vi "Teleop.vi"(10 "Match Info":T2={"Autonomous Elapsed Seconds"=0.0, "TeleOp Elapsed Seconds"=0.0, "Disabled Elapsed Seconds"=0.0, "Visited Autonomous"=FALSE, "Visited TeleOp"=FALSE, "Visited Disabled"=FALSE, "Autonomous Settings"={"Autonomous Style"=enum."Independent", "VI Refnum"=refnum}}, 11 "Call Context":T3) -> ()   [LabVIEW 2014]
doc: "This VI is called for each TeleOp packet received from the DS where the robot is not disabled. It is often used to read from the joysticks and update I/O or to update setpoints for timed control loops. It should complete and return within 20 milliseconds or it may miss DS packets."
uses:
  <vilib>/Rock Robotics/WPI/DriverStation/WPI_DriverStationDerivedRobotMode.ctl
  <vilib>/Rock Robotics/WPI/DriverStation/WPI_DriverStationMatch Info.ctl
  <vilib>/Rock Robotics/Network Tables/SD Read Boolean.vi
  <vilib>/Rock Robotics/Network Tables/SD Read Number.vi
  Robot Global Data.vi
  <vilib>/Rock Robotics/Network Tables/SD Write Numeric Array.vi
panel:
  out "Normalized Rect":T1
  out "Center":cluster{dbl, dbl}
  out "Applied Throttle":dbl
  out "Val":dbl
  out "RawVal":i32
  out "Stopped?":string
  out "Direction":string
  out "Distance":dbl
  out "Sample Slider 0":dbl(slide) scale=0.0..5.0
  out "Sample Boolean 1":bool
  out "Sample Boolean 0":bool
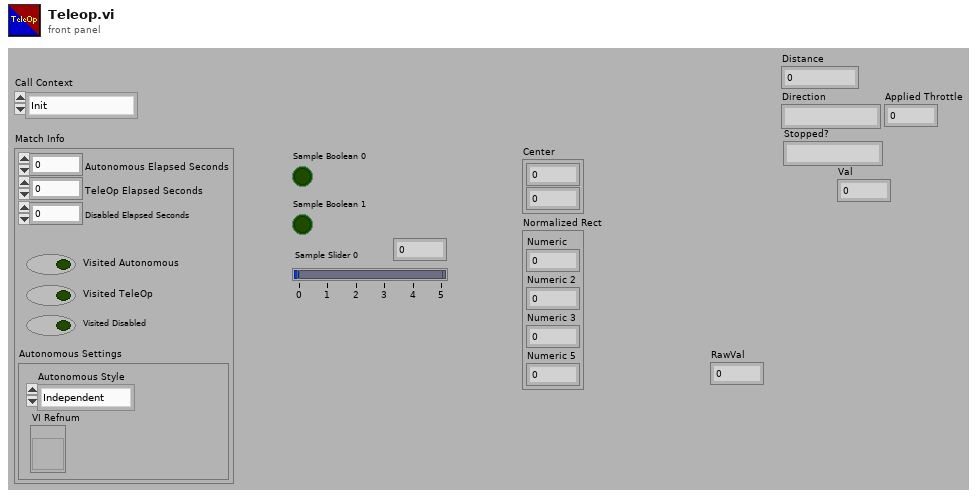
[diagram p1: front panel]
types:
  T1 = cluster{"Numeric":dbl, "Numeric 2":dbl, "Numeric 3":dbl, "Numeric 5":dbl}
  T2 = typedef "WPI_DriverStationMatch Info.ctl" = cluster{"Autonomous Elapsed Seconds":dbl, "TeleOp Elapsed Seconds":dbl, "Disabled Elapsed Seconds":dbl, "Visited Autonomous":bool, "Visited TeleOp":bool, "Visited Disabled":bool, "Autonomous Settings":cluster{"Autonomous Style":enum16{"Iterative", "Independent"}, "VI Refnum":refnum<vi>}}
  T3 = typedef "WPI_DriverStationDerivedRobotMode.ctl" = enum16{"Init", "Execute", "Stop"}
  T4 = typedef "WPI_MotorControlDeviceRef.ctl" = cluster{"DeviceStatus":errorcluster, "Type":T5, "PWM":cluster{"Controller":T6, "PWM Channel":T7, "DeadBand":T8}, "CAN":cluster{"Device Number":u8, "Control Mode":T9, "Semaphore":T10, "Max Vout":dbl, "TalonSRX Control Mode":T11}, "Invert":bool, "TransformRef":T12, "InvTransformRef":T12}
  T5 = typedef "WPI_MotorControlType.ctl" = enum16{"PWM", "CAN", "CANTalonSRX"}
  T6 = typedef "FPGA_TypedefDigitalModule.ctl" = enum16{"Controller 1"}
  T7 = typedef "FPGA_DIOPWMChannel.ctl" = enum8{"PWM 0", "PWM 1", "PWM 2", "PWM 3", "PWM 4", "PWM 5", "PWM 6", "PWM 7", "PWM 8", "PWM 9", "PWM MXP 0", "PWM MXP 1", "PWM MXP 2", "PWM MXP 3", "PWM MXP 4", "PWM MXP 5", "PWM MXP 6", "PWM MXP 7", "PWM MXP 8", "PWM MXP 9", "Invalid"}
  T8 = typedef "WPI_PWMDeadband.ctl" = cluster{"Name":string, "maxPositivePwm":i32, "minPositivePwm":i32, "centerPwm":i32, "maxNegativePwm":i32, "minNegativePwm":i32, "angularRange":u16}
  T9 = typedef "WPI_CANJaguar_ControlMode.ctl" = enum8{"Percent VBus", "Current", "Speed", "Position", "Voltage"}
  T10 = typedef "Semaphore RefNum" = refnum<k1>
  T11 = typedef "WPI_CANTalonSRX_APIControlMode.ctl" = enum8{"Percent VBus", "Speed", "Position", "Slave", "Unchanged / Invalid"}
  T12 = typedef "WPI_PWMTransform_ConPane.ctl" = refnum<vi>
  T13 = typedef "WPI_CANTalonSRX_GlobalStatus.ctl" = cluster{"Applied Throttle":dbl, "Module Enabled":bool, "CAN Error":errorcluster, "Closed Loop Error":dbl, "Forward Limit Switch Closed":bool, "Reverse Limit Switch Closed":bool, "Sensor Position":dbl, "Sensor Velocity":dbl, "Current":dbl, "Sticky Fault - Over Temp":bool, "Sticky Fault - Under Voltage":bool, "Sticky Fault - Forward Limit":bool, "Sticky Fault - Reverse Limit":bool, "Sticky Fault - Forward Soft Limit":bool, "Sticky Fault - Reverse Soft Limit":bool, "Brake is Enabled":bool, "Encoder Position":dbl, "Encoder Velocity":dbl, "Encoder Index Count":dbl, "Encoder A Pin State":bool, "Encoder B Pin State":bool, "Encoder Index Pin State":bool, "Analog In":dbl, "Analog In Velocity":dbl, "Temperature (C)":dbl, "Battery Voltage":dbl}
  T14 = cluster{"Distance (ft)":dbl, "Center":cluster{dbl, dbl}, "Normalized Rect":cluster{"Numeric":dbl, "Numeric 2":dbl, "Numeric 3":dbl, "Numeric 5":dbl}}[]
  T15 = cluster{"Detected Totes[0]":cluster{"Distance (ft)":dbl, "Center":cluster{dbl, dbl}, "Normalized Rect":cluster{"Numeric":dbl, "Numeric 2":dbl, "Numeric 3":dbl, "Numeric 5":dbl}}, "Detected Totes[1]":cluster{"Distance (ft)":dbl, "Center":cluster{dbl, dbl}, "Normalized Rect":cluster{"Numeric":dbl, "Numeric 2":dbl, "Numeric 3":dbl, "Numeric 5":dbl}}, "Detected Totes[2]":cluster{"Distance (ft)":dbl, "Center":cluster{dbl, dbl}, "Normalized Rect":cluster{"Numeric":dbl, "Numeric 2":dbl, "Numeric 3":dbl, "Numeric 5":dbl}}, "Detected Totes[3]":cluster{"Distance (ft)":dbl, "Center":cluster{dbl, dbl}, "Normalized Rect":cluster{"Numeric":dbl, "Numeric 2":dbl, "Numeric 3":dbl, "Numeric 5":dbl}}, "Detected Totes[4]":cluster{"Distance (ft)":dbl, "Center":cluster{dbl, dbl}, "Normalized Rect":cluster{"Numeric":dbl, "Numeric 2":dbl, "Numeric 3":dbl, "Numeric 5":dbl}}, "Detected Totes[5]":cluster{"Distance (ft)":dbl, "Center":cluster{dbl, dbl}, "Normalized Rect":cluster{"Numeric":dbl, "Numeric 2":dbl, "Numeric 3":dbl, "Numeric 5":dbl}}, "Detected Totes[6]":cluster{"Distance (ft)":dbl, "Center":cluster{dbl, dbl}, "Normalized Rect":cluster{"Numeric":dbl, "Numeric 2":dbl, "Numeric 3":dbl, "Numeric 5":dbl}}, "Detected Totes[7]":cluster{"Distance (ft)":dbl, "Center":cluster{dbl, dbl}, "Normalized Rect":cluster{"Numeric":dbl, "Numeric 2":dbl, "Numeric 3":dbl, "Numeric 5":dbl}}, "Detected Totes[8]":cluster{"Distance (ft)":dbl, "Center":cluster{dbl, dbl}, "Normalized Rect":cluster{"Numeric":dbl, "Numeric 2":dbl, "Numeric 3":dbl, "Numeric 5":dbl}}}
  T16 = cluster{"Distance (ft)":dbl, "Center":cluster{dbl, dbl}, "Normalized Rect":cluster{"Numeric":dbl, "Numeric 2":dbl, "Numeric 3":dbl, "Numeric 5":dbl}}
  T17 = typedef "WPI_EncoderDevRef.ctl" = cluster{"DevStatus":errorcluster, "EncoderIndex":T18, "CounterIndex":T19, "DistancePerCount":dbl, "Decoding Type":T20}
  T18 = typedef "FPGA_EncoderIdx.ctl" = enum8{"Enc 0", "Enc 1", "Enc 2", "Enc 3", "Enc 4", "Enc 5", "Enc 6", "Enc 7", "Invalid"}
  T19 = typedef "FPGA_CounterCtrSystemIndex.ctl" = enum8{"Ctr 0", "Ctr 1", "Ctr 2", "Ctr 3", "Ctr 4", "Ctr 5", "Ctr 6", "Ctr 7", "Invalid"}
  T20 = typedef "WPI_EncoderType.ctl" = enum16{"1x", "2x", "4x"}
  T21 = typedef "WPI_CounterDevRef.ctl" = cluster{"DevStatus":errorcluster, "CntIndex":T19}
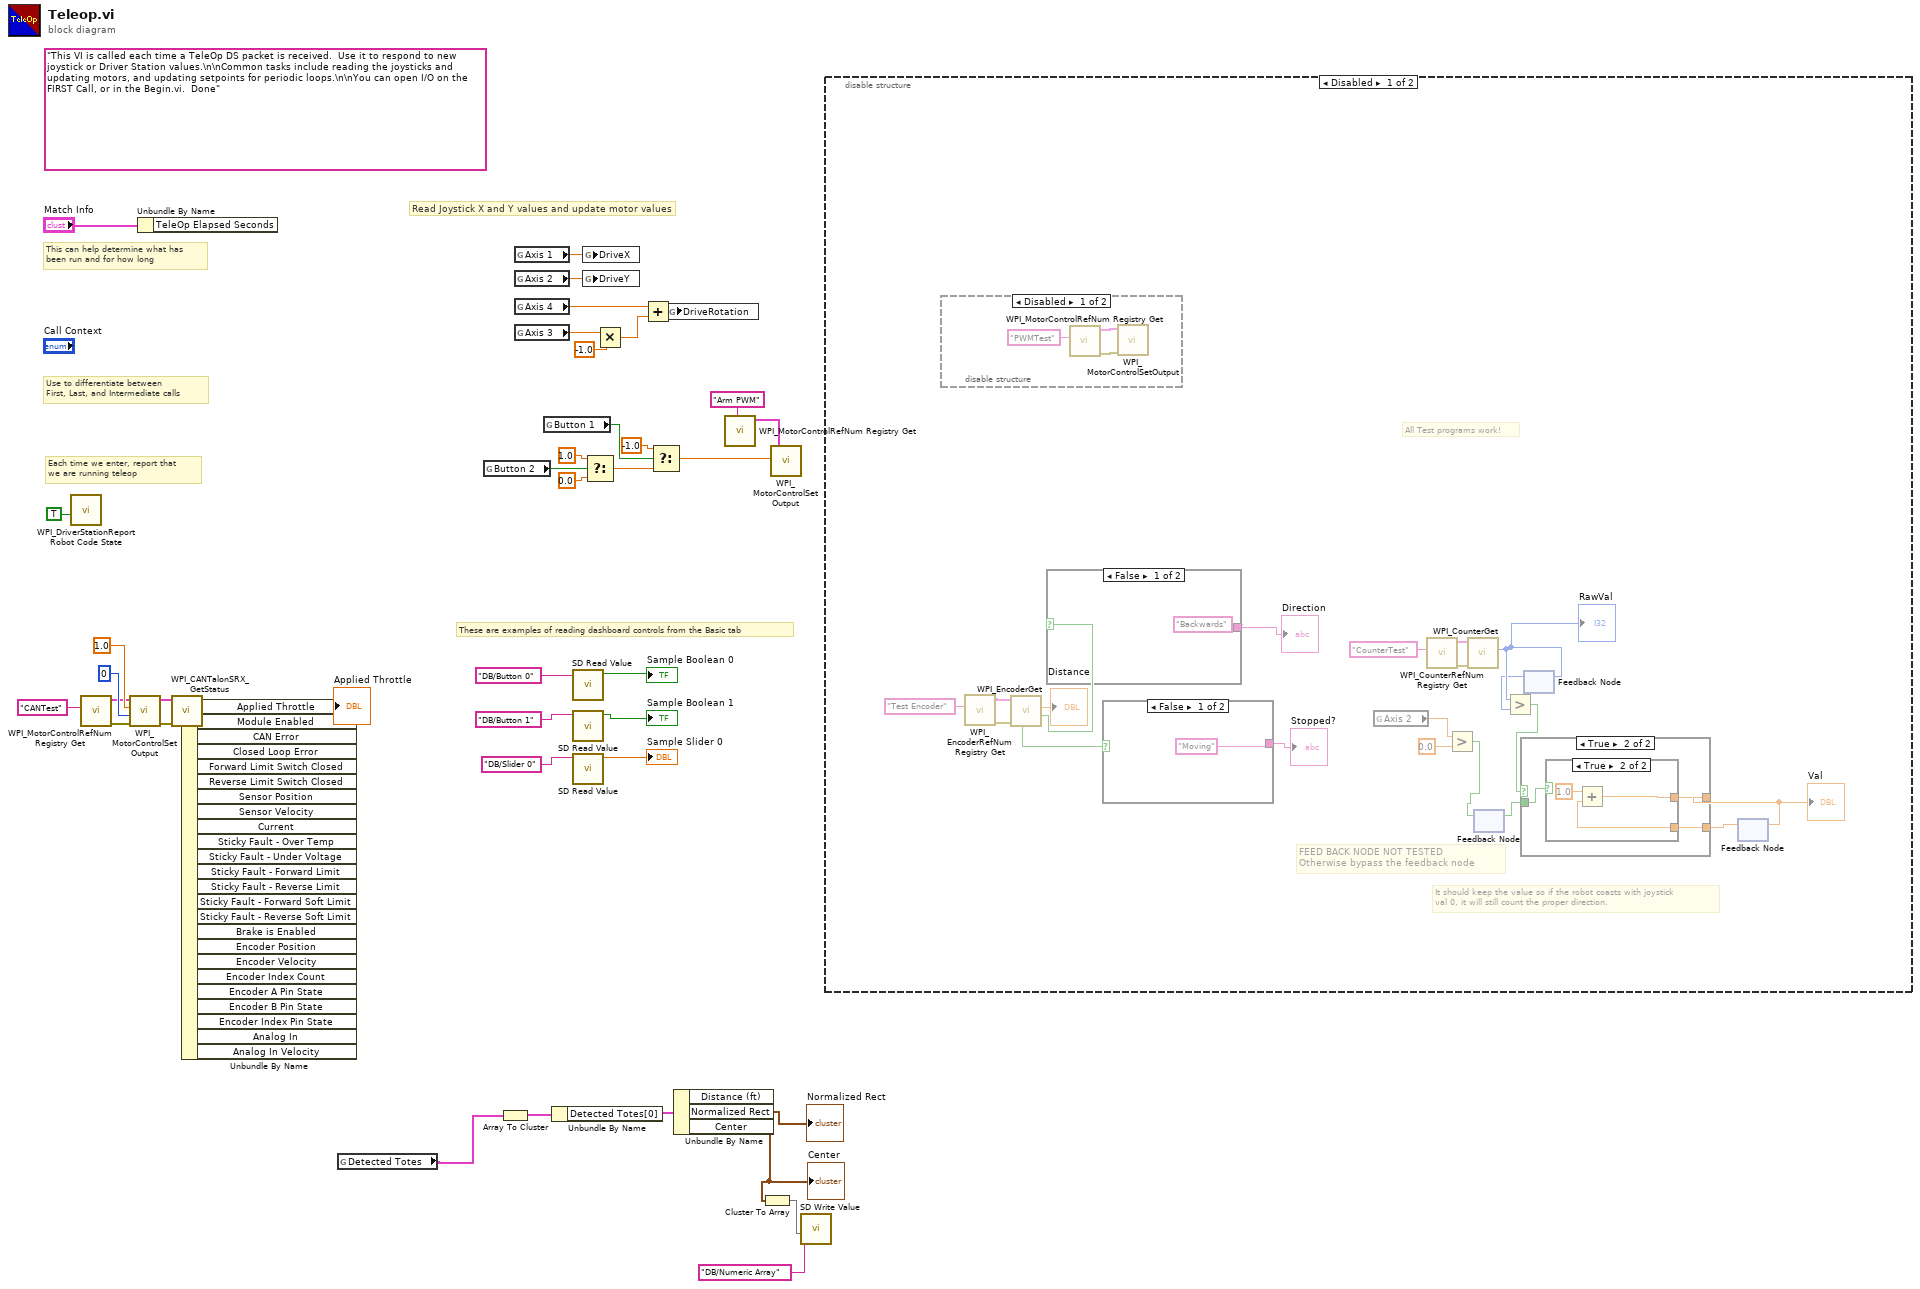
[diagram p0: block diagram]
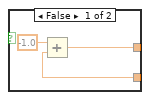
[diagram p4: hidden frame]
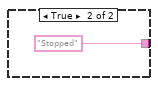
[diagram p5: hidden frame]
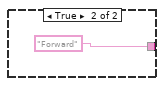
[diagram p6: hidden frame]
diagram:
  (unwired) "This VI is called each time a TeleOp DS packet is received.  Use it to respond to new joystick or Driver Station values.\n\nCommon tasks include reading the joysticks and updating motors, and updating setpoints for periodic loops.\n\nYou can open I/O on the FIRST Call, or in the Begin.vi.  Done"
  # "These are examples of reading dashboard controls from the Basic tab"
  # "Each time we enter, report that\nwe are running teleop"
  # "Use to differentiate between\nFirst, Last, and Intermediate calls"
  # "This can help determine what has\nbeen run and for how long"
  # "Read Joystick X and Y values and update motor values"
  n1 = call <vilib>:"WPI_DriverStationReport Robot Code State.vi"("TeleOp"=TRUE ("Autonomous")) -> ()  [unwired: 10 in, 1 out]
  n2 = call <vilib>:"WPI_MotorControlRefNum Registry Get.vi"("refnum name"="CANTest") -> ("error out"=w9:errorcluster, "MotorControlDevRef"=w8:T4)  [unwired: 9 in]
  n3 = call <vilib>:"WPI_MotorControlSetOutput.vi"("error in (no error)"=w9, "Sync Group / Parameter Slot"=u8 0, "Output"=1.0, "MotorControlDevRef"=w8) -> ("error out"=w12:errorcluster, "MotorControlDevRef"=w13:T4)  [unwired: 5 in, 1 out]
  n4 = Unbundle By Name("Match Info") -> ()  [unwired: 1 out]
  n5 = call <vilib>:"WPI_CANTalonSRX_GetStatus.vi"("error in (no error)"=w12, "CAN Talon SRX Ref"=w13) -> ("Talon SRX Status"=w14:T13)  [unwired: 7 in, 2 out]
  n6 = Unbundle By Name(w14) -> ("Applied Throttle"=→"Applied Throttle":dbl)  [unwired: 23 out]
  n7 = global read "Robot Global Data.vi" "Detected Totes"() -> (w5:T14)
  n8 = global read "Robot Global Data.vi" "Button 2"() -> (w19:bool)
  n9 = Array To Cluster(array=w5) -> (cluster=w7:T15)
  n10 = global read "Robot Global Data.vi" "Axis 1"() -> (w27:dbl)
  n11 = global read "Robot Global Data.vi" "Axis 2"() -> (w26:dbl)
  n12 = global read "Robot Global Data.vi" "Axis 4"() -> (w22:dbl)
  n13 = global read "Robot Global Data.vi" "Axis 3"() -> (w23:dbl)
  n14 = global read "Robot Global Data.vi" "Button 1"() -> (w20:bool)
  n15 = Unbundle By Name(w7) -> ("Detected Totes[0]"=w6:T16)
  n16 = call-poly <vilib>:"SD Read Value.vi"("Name"="DB/Button 0" ("refnum name")) -> ("Boolean"=→"Sample Boolean 0":bool)  [unwired: 8 in, 2 out]
  n17 = call-poly <vilib>:"SD Read Value.vi"("Name"="DB/Button 1" ("refnum name")) -> ("Boolean"=→"Sample Boolean 1":bool)  [unwired: 8 in, 2 out]
  n18 = call-poly <vilib>:"SD Read Value.vi"("Name"="DB/Slider 0" ("refnum name")) -> ("Numeric"=→"Sample Slider 0":dbl)  [unwired: 8 in, 2 out]
  n19 = global write "Robot Global Data.vi" "DriveX"(w27) -> ()
  n20 = global write "Robot Global Data.vi" "DriveY"(w26) -> ()
  n21 = Select(t=1.0, s=w19, f=0.0) -> (s? t:f=w30:dbl)
  n22 = Multiply(x=w23, y=-1.0) -> (x*y=w24:dbl)
  n23 = Add(x=w22, y=w24) -> (x+y=w21:dbl)
  n24 = Select(t=-1.0, s=w20, f=w30) -> (s? t:f=w28:dbl)
  n25 = global write "Robot Global Data.vi" "DriveRotation"(w21) -> ()
  n26 = Unbundle By Name(w6) -> ("Normalized Rect"=→"Normalized Rect":T1, "Center"=w3:cluster{dbl, dbl})  [unwired: 1 out]
  "Center" <- w3
  n27 = call <vilib>:"WPI_MotorControlRefNum Registry Get.vi"("refnum name"="Arm PWM") -> ("MotorControlDevRef"=w17:T4)  [unwired: 9 in, 1 out]
  n28 = Cluster To Array(cluster=w3) -> (array=w2:dbl[])
  n29 = call <vilib>:"WPI_MotorControlSetOutput.vi"("Output"=w28, "MotorControlDevRef"=w17) -> ()  [unwired: 7 in, 3 out]
  n30 = call-poly <vilib>:"SD Write Value.vi"("Numeric Array"=w2, "Name"="DB/Numeric Array") -> ()  [unwired: 8 in, 2 out]
  n31 = disable-structure shown="Disabled" {
    frame Disabled {
      # "It should keep the value so if the robot coasts with joystick\nval 0, it will still count the proper direction."
      # "All Test programs work!"
      # "FEED BACK NODE NOT TESTED\nOtherwise bypass the feedback node"
      n32 = disable-structure shown="Disabled" {
        frame Disabled {
          n33 = call <vilib>:"WPI_MotorControlRefNum Registry Get.vi"("refnum name"="PWMTest") -> ("error out"=w62:errorcluster, "MotorControlDevRef"=w63:T4)  [unwired: 9 in]
          n34 = call <vilib>:"WPI_MotorControlSetOutput.vi"("error in (no error)"=w62, "MotorControlDevRef"=w63) -> ()  [unwired: 7 in, 3 out]
        }
        frame Enabled {
        }
      }
      n35 = call <vilib>:"WPI_EncoderRefNum Registry Get.vi"("refnum name"="Test Encoder") -> ("error out"=w58:errorcluster, "EncoderDevRef"=w59:T17)  [unwired: 9 in]
      n36 = call <vilib>:"WPI_EncoderGet.vi"("error in (no error)"=w58, "EncoderDevRef"=w59) -> ("Direction"=w55:bool, "Distance"=→"Distance":dbl, "Stopped"=w54:bool)  [unwired: 4 in, 3 out]
      n37 = case shown="False" w55 {
        tunnel: ["Backwards" "Forward"] -> w56
        frame False {
        }
        frame True {
        }
      }
      "Direction" <- w56
      n38 = case shown="False" w54 {
        tunnel: ["Moving" "Stopped"] -> w53
        frame False {
        }
        frame True {
        }
      }
      "Stopped?" <- w53
      n39 = global read "Robot Global Data.vi" "Axis 2"() -> (w41:dbl)
      n40 = call <vilib>:"WPI_CounterRefNum Registry Get.vi"("refnum name"="CounterTest") -> ("error out"=w51:errorcluster, "CounterDevRef"=w50:T21)  [unwired: 9 in]
      n41 = Greater?(x=w41, y=0.0) -> (0:w43:bool)
      n42 = call <vilib>:"WPI_CounterGet.vi"("error in (no error)"=w51, "CounterDevRef in"=w50) -> ("Value"=w48:i32)  [unwired: 4 in, 5 out]
      "RawVal" <- w48
      n43 = feedback #1() -> (w42:bool)  [unwired: 1 in]
      n44 = feedback-in #1(w43) -> ()
      n45 = feedback #2() -> (w47:i32)  [unwired: 1 in]
      n46 = Greater?(x=w48, y=w47) -> (0:w46:bool)
      n47 = feedback-in #2(w48) -> ()
      n48 = feedback #3() -> (w44:dbl)  [unwired: 1 in]
      n49 = case shown="True" w46 {
        tunnel: w42 -> [_ w65]
        tunnel: [w64 w67] -> w45
        tunnel: w44 -> [w64 w66]
        frame False {
        }
        frame True {
          n50 = case shown="True" w65 {
            tunnel: [w69 w72] -> w67
            tunnel: w66 -> [w68 w71]
            frame False {
              n51 = Add(x=-1.0, y=w68) -> (x+y=w69:dbl)
            }
            frame True {
              n52 = Add(x=1.0, y=w71) -> (x+y=w72:dbl)
            }
          }
        }
      }
      "Val" <- w45
      n53 = feedback-in #3(w45) -> ()
    }
    frame Enabled {
    }
  }
